vi "Select Channel.vi"(8 "error in (no error)":errorcluster, 10 "Channel":i32, 11 "LR-700 Driver in":refnum<class "LR-700 Driver.lvclass">) -> (0 "error out":errorcluster, 3 "LR-700 Driver out":refnum<class "LR-700 Driver.lvclass">)   [LabVIEW 2019, in "LR-700 Driver.lvclass"]
uses:
  LR-700 Driver.lvclass
  C:/GitHub/NHMFL_Core/Libraries/Instruments/VISA Instrument/VISA Instrument.lvclass
  VISA Instrument/VISA Instrument.lvclass/VISA Instrument.ctl
  VISA Instrument/Read VISA resource.vi
  VISA Instrument/Write VISA resource.vi
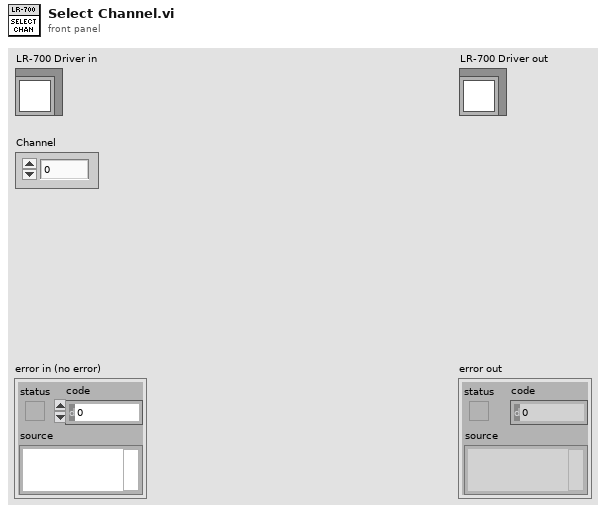
[diagram p1: front panel]
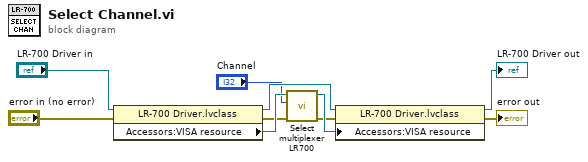
[diagram p0: block diagram]
diagram:
  n1 = property class="LR-700 Driver.lvclass"(reference="LR-700 Driver in", error in="error in (no error)") -> (reference out=w8:refnum<class "LR-700 Driver.lvclass">, error out=w2:errorcluster, "Accessors:VISA resource"=w5:refnum<visa-resource-name>)
  n2 = call "Select multiplexer LR700.vi"("error in"=w2, "Sensor"="Channel", "VISA Resource Name"=w5) -> ("error out"=w1:errorcluster, "VISA Resource Name Out"=w4:refnum<visa-resource-name>)  [unwired: 7 in]
  n3 = property class="LR-700 Driver.lvclass"(reference=w8, error in=w1, "Accessors:VISA resource"=w4) -> (reference out=→"LR-700 Driver out":refnum<class "LR-700 Driver.lvclass">, error out=→"error out":errorcluster)
